vi "1d Median Filter.vi"(9 "Filter Width":i32, 11 "Unfiltered Data":dbl[](array[numeric])) -> (3 "Median Filtered data out":dbl[](array[numeric]))   [LabVIEW 2013]
doc: "Runs a median filter on windowed 1d array (dbl)"
uses:
  <vilib>/Analysis/NI_AALBase.lvlib
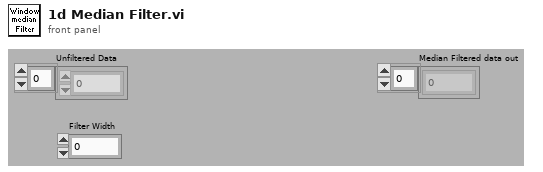
[diagram p1: front panel]
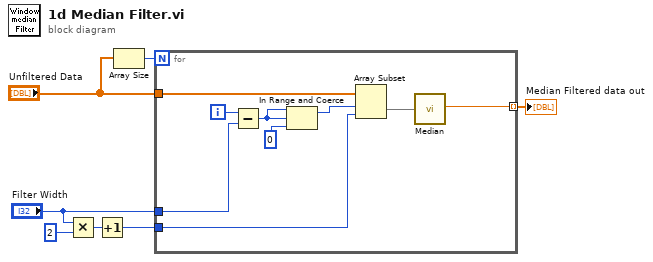
[diagram p0: block diagram]
diagram:
  n1 = Multiply(x="Filter Width", y=2) -> (x*y=w5:i32)
  n2 = Increment(x=w5) -> (x+1=w4:i32)
  n3 = Array Size(array="Unfiltered Data") -> (size(s)=w2:i32)
  n4 = for {
    N: w2 -> [_]
    tunnel: "Unfiltered Data" -> [w16]
    tunnel: "Filter Width" -> [w14]
    tunnel: w4 -> [w10]
    tunnel: [w8] -> w3 mode=indexing
    i -> [w15]
    n5 = Subtract(x=w15, y=w14) -> (x-y=w13:i32)
    n6 = In Range and Coerce(upper limit=w13, x=w13, lower limit=0) -> (coerced(x)=w11:i32)  [unwired: 1 out]
    n7 = Array Subset(array=w16, index=w11, length=w10) -> (w9:dbl[])
    n8 = call <vilib>:"Median.vi"("X"=w9) -> ("median"=w8:dbl)  [unwired: 1 out]
  }
  "Median Filtered data out" <- w3
